vi "serialComm.vi"(8 "error in (no error)":errorcluster, 10 "write buffer":string, 11 "VISA resource name":refnum<visa-resource-name>) -> (0 "error out":errorcluster, 2 "read buffer":string, 3 "VISA resource name 2":refnum<visa-resource-name>)   [LabVIEW 2012]
uses:
  <vilib>/regexp/Match Regular Expression.xnode
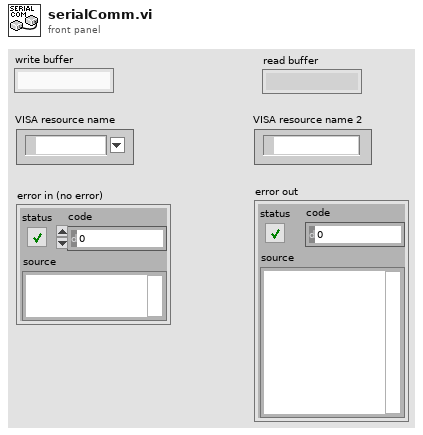
[diagram p1: front panel]
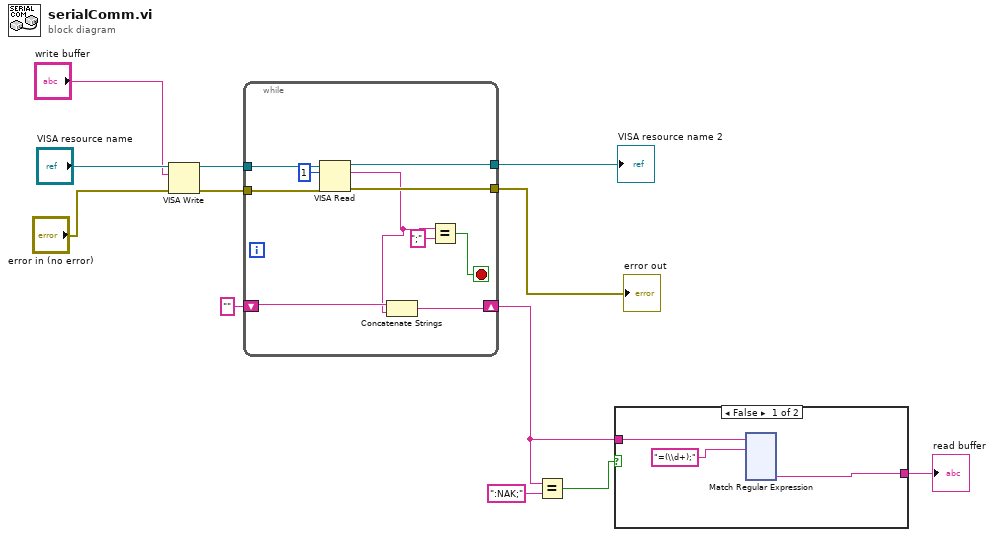
[diagram p0: block diagram]
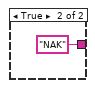
[diagram p2: hidden frame]
diagram:
  n1 = VISA Write(VISA resource name="VISA resource name", write buffer="write buffer", error in (no error)="error in (no error)") -> (VISA resource name out=w3:refnum<visa-resource-name>, error out=w10:errorcluster)  [unwired: 1 out]
  n2 = while {
    tunnel: w10 -> [w22]
    tunnel: [w21] -> w8
    tunnel: [w20] -> w7
    tunnel: w3 -> [w19]
    shift-right: [w16] -> w2
    shift-left: "" -> [w15]
    stop <- w18 stop-if-true
    n3 = VISA Read(VISA resource name=w19, byte count=u32 1, error in (no error)=w22) -> (VISA resource name out=w21:refnum<visa-resource-name>, read buffer=w14:string, error out=w20:errorcluster)  [unwired: 1 out]
    n4 = Concatenate Strings(w15, w14) -> (w16:string)
    n5 = Equal?(x=w14, y=";") -> (x = y?=w18:bool)
  }
  "VISA resource name 2" <- w8
  "error out" <- w7
  n6 = Equal?(x=w2, y=":NAK;") -> (x = y?=w5:bool)
  n7 = case shown="False" w5 {
    tunnel: w2 -> [w24 _]
    tunnel: [w23 "NAK" ("submatch 1")] -> w4
    frame False {
      n8 = xnode "Match Regular Expression"("input string"=w24, "regular expression"="=(\\d+);") -> ("submatch 1"=w23:string)  [unwired: 4 in, 5 out]
    }
    frame True {
    }
  }
  "read buffer" <- w4
